vi "BCC校验码.vi"(11 "指令内容":string) -> (0 "最终内容":string, 3 "校验码":string)   [LabVIEW 8.6]
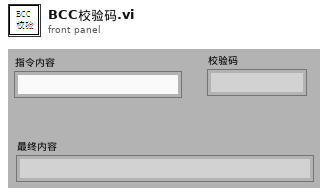
[diagram p1: front panel]
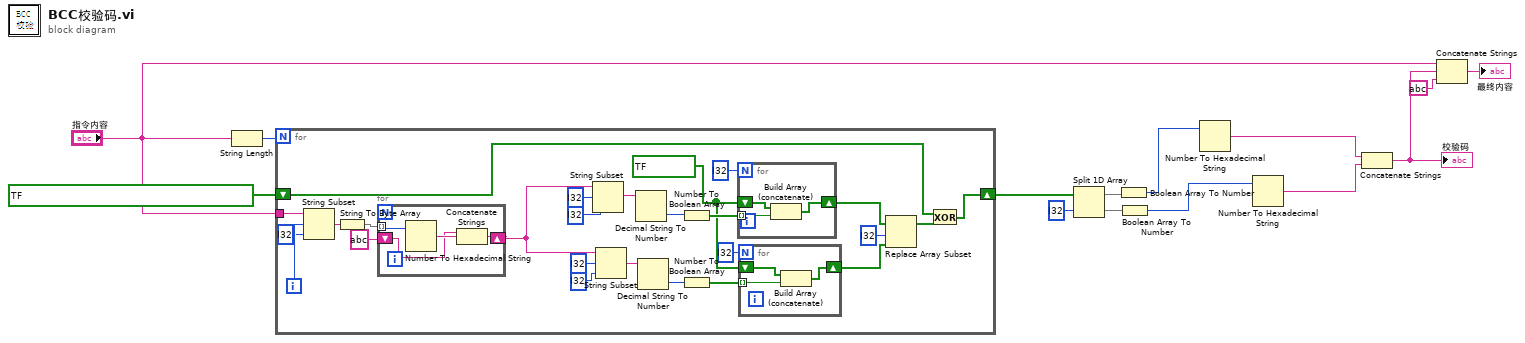
[diagram p0: block diagram]
diagram:
  n1 = String Length(string="指令内容") -> (length=w9:i32)
  n2 = for {
    N: w9 -> [_]
    tunnel: "指令内容" -> [w40]
    shift-right: [w20] -> w13
    shift-left: bool[] ? -> [w19]
    i -> [w39]
    w24 = bool[] ?
    n3 = String Subset(string=w40, offset (0)=w39, length (rest)=i32 ? ("length (rest)")) -> (substring=w18:string)
    n4 = String To Byte Array(string=w18) -> (unsigned byte array=w17:u8[])
    n5 = for {
      tunnel: w17 -> [w44] mode=indexing
      shift-right: [w42] -> w16
      shift-left: string ? -> [w41]
      n6 = Number To Hexadecimal String(2:w44) -> (0:w43:string)  [unwired: 1 in]
      n7 = Concatenate Strings(w41, w43) -> (w42:string)
    }
    n8 = String Subset(string=w16, offset (0)=i32 ?, length (rest)=i32 ? ("length (rest)")) -> (substring=w33:string)
    n9 = String Subset(string=w16, offset (0)=i32 ?, length (rest)=i32 ? ("length (rest)")) -> (substring=w32:string)
    n10 = Decimal String To Number(string=w33) -> (number=w31:i32)  [unwired: 2 in, 1 out]
    n11 = Decimal String To Number(string=w32) -> (number=w30:i32)  [unwired: 2 in, 1 out]
    n12 = Number To Boolean Array(number=w31) -> (Boolean array=w29:bool[])
    n13 = Number To Boolean Array(number=w30) -> (Boolean array=w25:bool[])
    n14 = for {
      N: i32 ? -> [_]
      tunnel: w29 -> [w50] mode=indexing
      shift-right: [w48] -> w27
      shift-left: w24 -> [w49]
      n15 = Build Array (concatenate)(w49, w50) -> (w48:bool[])
    }
    n16 = for {
      N: i32 ? -> [_]
      tunnel: w25 -> [w47] mode=indexing
      shift-right: [w45] -> w23
      shift-left: w24 -> [w46]
      n17 = Build Array (concatenate)(w46, w47) -> (w45:bool[])
    }
    n18 = Replace Array Subset(array=w27, new element=w23, index=i32 ?) -> (w21:bool[])
    n19 = Exclusive Or(1:w21, 2:w19) -> (0:w20:bool[])
  }
  n20 = Split 1D Array(array=w13, index=i32 ?) -> (first subarray=w11:bool[], second subarray=w10:bool[])
  n21 = Boolean Array To Number(Boolean array=w11) -> (number=w8:u32)
  n22 = Boolean Array To Number(Boolean array=w10) -> (number=w7:u32)
  n23 = Number To Hexadecimal String(2:w8) -> (0:w4:string)  [unwired: 1 in]
  n24 = Number To Hexadecimal String(2:w7) -> (0:w3:string)  [unwired: 1 in]
  n25 = Concatenate Strings(w4, w3) -> (w6:string)
  "校验码" <- w6
  n26 = Concatenate Strings("指令内容", w6, string ?) -> (→"最终内容":string)
